vi "Get Identifier.vi"(8 "Error In":errorcluster, 11 "Communicator in":refnum<class "Communicator.lvclass">) -> (0 "Error Out":errorcluster, 2 "Identifier":string, 3 "Communicator out":refnum<class "Communicator.lvclass">)   [LabVIEW 2024, in "Communicator.lvclass"]
uses:
  Communicator.lvclass
  Communicator.lvclass/Communicator.ctl
  Interfaces/IConfigure/IConfigure.lvclass
  Interfaces/IConfiguration/IConfiguration.lvclass
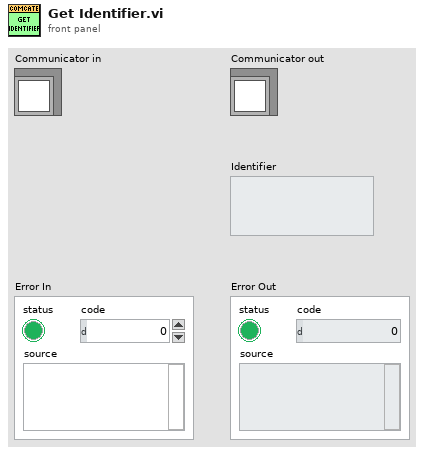
[diagram p1: front panel]
types:
  T1 = typedef "Communicator.lvclass/ObjectAttributes.ctl" = cluster{"IConfigure":refnum<class "IConfigure.lvclass">, "Worker Enqueuer":refnum<class "Message Enqueuer.lvclass">}
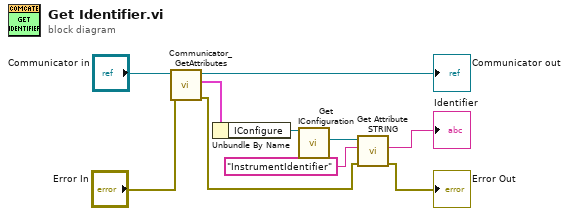
[diagram p0: block diagram]
diagram:
  n1 = call "Communicator_GetAttributes.vi"("Error In"="Error In", "Communicator in"="Communicator in") -> ("Error Out"=w2:errorcluster, "Data"=w6:T1, "Communicator out"=→"Communicator out":refnum<class "Communicator.lvclass">)  [unwired: 6 in, 1 out]
  n2 = Unbundle By Name(w6) -> ("IConfigure"=w5:refnum<class "IConfigure.lvclass">)
  n3 = call-dynamic "Get IConfiguration.vi"("IConfigure in"=w5) -> ("IConfiguration"=w4:refnum<class "IConfiguration.lvclass">)  [unwired: 9 in, 1 out]
  n4 = call-dynamic "Get Attribute STRING.vi"("error in"=w2, "Attribute"="InstrumentIdentifier", "IConfiguration in"=w4) -> ("error out"=→"Error Out":errorcluster, "Value"=→"Identifier":string)  [unwired: 6 in, 1 out]
